vi "接收.vi"(8 "error in (no error)":errorcluster caption="错误输入（无错误）", 11 "VISA 输入":refnum<class "VISA.lvclass">) -> (0 "error out":errorcluster caption="错误输出", 2 "消息类.lvclass":refnum<class "消息类.lvclass">, 3 "VISA 输出":refnum<class "VISA.lvclass">)   [LabVIEW 2016, in "VISA.lvclass"]
uses:
  VISA.lvclass
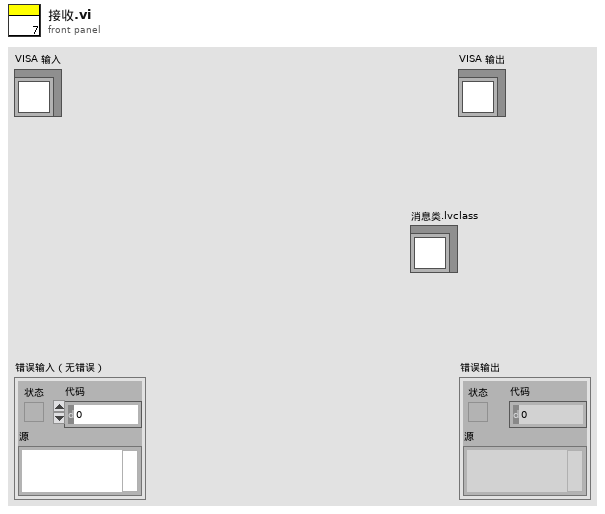
[diagram p1: front panel]
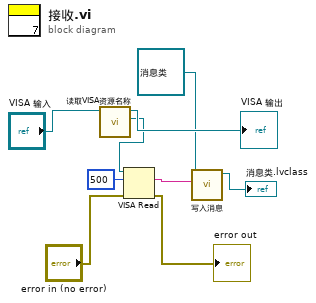
[diagram p0: block diagram]
diagram:
  n1 = call-dynamic "读取VISA资源名称.vi"("VISA输入"="VISA 输入") -> ("VISA资源名称"=w7:refnum<visa-resource-name>, "VISA输出"=→"VISA 输出":refnum<class "VISA.lvclass">)  [unwired: 8 in, 1 out]
  n2 = VISA Read(VISA resource name=w7, byte count=u32 500 ("字节总数"), error in (no error)="error in (no error)") -> (read buffer=w3:string, error out=→"error out":errorcluster)  [unwired: 2 out]
  n3 = call-dynamic "写入消息.vi"("消息"=w3, "消息类输入"=refnum<class "消息类.lvclass"> refnum ("消息类.lvclass")) -> ("消息类输出"=→"消息类.lvclass":refnum<class "消息类.lvclass">)  [unwired: 8 in, 1 out]
